vi "DRAWING_TREE_INDI.vi"(7 "Array":string[](array[string]), 8 "error in (no error)":errorcluster, 9 "NewVal":string, 10 "Array 2":string[](array[string]), 11 "TreeControl in":refnum<vi>) -> (0 "error out":errorcluster)   [LabVIEW 2017]
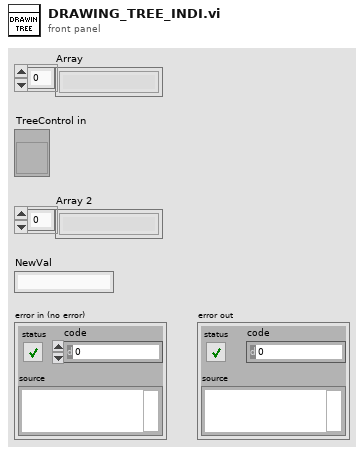
[diagram p1: front panel]
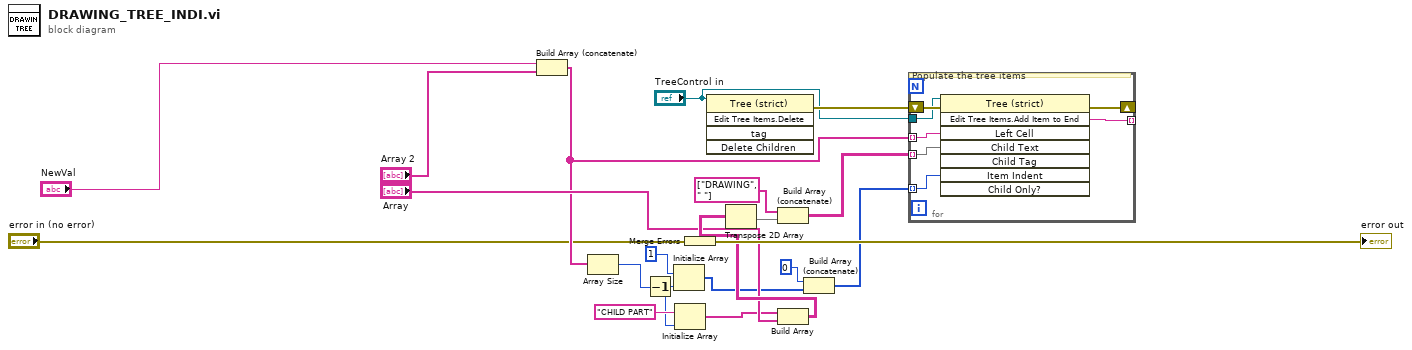
[diagram p0: block diagram]
diagram:
  n1 = Build Array (concatenate)("NewVal", "Array 2") -> (w8:string[])
  n2 = Array Size(array=w8) -> (size(s)=w9:i32)
  n3 = Decrement(x=w9) -> (x-1=w14:i32)
  n4 = Initialize Array(1, w14) -> (w11:i32[])
  n5 = Initialize Array("CHILD PART" ("String"), w14) -> (w16:string[])
  n6 = Merge Errors("error in (no error)") -> (→"error out":errorcluster)
  n7 = invoke on="Invoke Node" class="Tree (strict)" method="Edit Tree Items.Delete"(reference="TreeControl in") -> (error out=w5:errorcluster)  [unwired: 4 in, 4 out]
  n8 = Build Array(w16, "Array") -> (w19:string[][])
  n9 = Transpose 2D Array(2D array=w19) -> (transposed array=w18:string[][])
  n10 = Build Array (concatenate)(string[] ["DRAWING", " "] ("First item attributes"), w18) -> (w3:string[][])
  n11 = Build Array (concatenate)(0, w11) -> (w12:i32[])
  n12 = for {
    tunnel: w8 -> [w26] mode=indexing
    tunnel: [w25] -> _ mode=indexing
    tunnel: w12 -> [w24] mode=indexing
    tunnel: w3 -> [w22] mode=indexing
    shift-right: [w23] -> _
    shift-left: w5 -> [w27]
    tunnel: "TreeControl in" -> [w21]
    # "Populate the tree items"
    n13 = invoke on="Invoke Node" class="Tree (strict)" method="Edit Tree Items.Add Item to End"(reference=w21, error in=w27, "Left Cell"=w26, "Child Text"=w22, "Item Indent"=w24) -> (error out=w23:errorcluster, "Edit Tree Items:Add Item to End"=w25:string)  [unwired: 3 in, 6 out]
  }
